vi "Read ADU Packet.vi"(8 "error in":errorcluster, 10 "isMaster (f)":bool, 11 "IP simple ADU in":refnum<class "SMSD ADU.lvclass">) -> (0 "error out":errorcluster, 2 "SMSD data unit out":refnum<class "SMSD Data Unit.lvclass">, 3 "IP simple ADU out":refnum<class "SMSD ADU.lvclass">, 5 "PDU Valid?":bool)   [LabVIEW 2021, in "SMSD ADU.lvclass"]
doc: "This uses the protocol layer to read a modbus packet off of the bus, wrapped in the IP transmission data unit."
uses:
  SMSD ADU.lvclass
  Data Unit/SMSD Data Unit/SMSD Data Unit.lvclass
  SMSD ADU.lvclass/SMSD ADU.ctl
  Data Unit/SMSD Data Unit/SMSD Data Unit.lvclass/SMSD Data Unit.ctl
  <vilib>/Utility/error.llb/Clear Errors.vi
  Modbus_v121c/Network Interface/TCP Interface/TSC/TCP Shared Components.lvlib
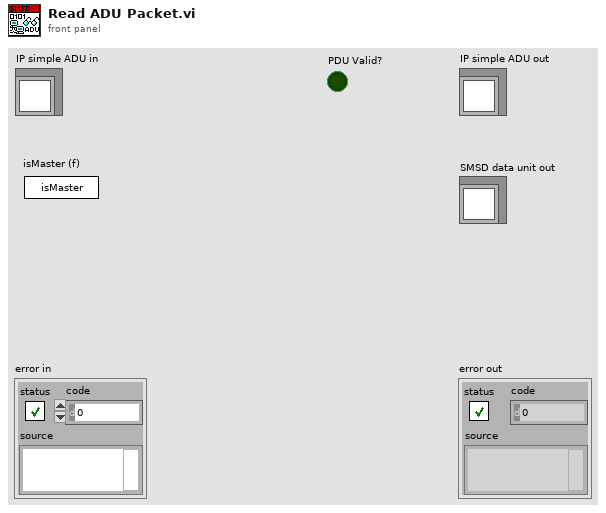
[diagram p1: front panel]
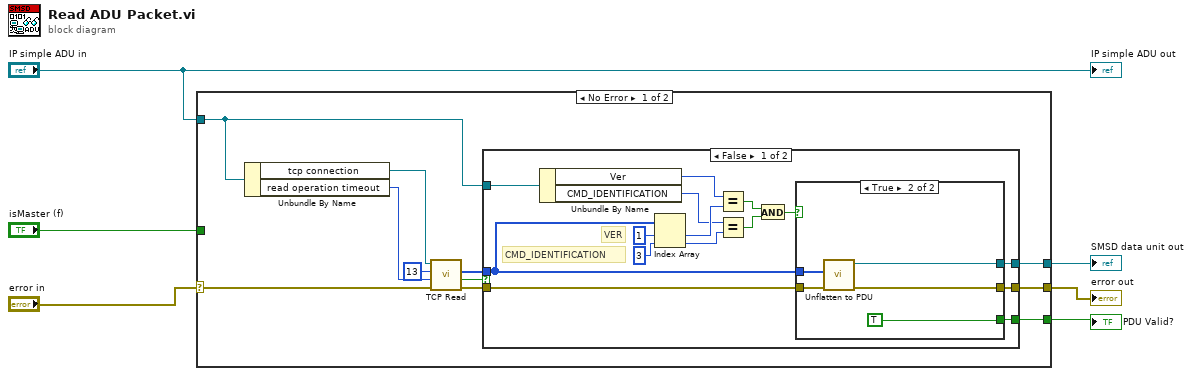
[diagram p0: block diagram]
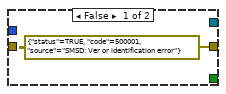
[diagram p2: hidden frame]
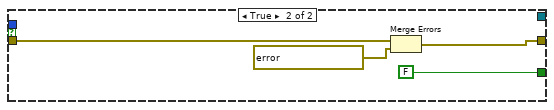
[diagram p3: hidden frame]
diagram:
  n1 = case shown="No Error" "error in" {
    selector: "error in" -> [w11 w43]
    tunnel: [w17 w43] -> w5
    tunnel: "IP simple ADU in" -> [w7 _]
    tunnel: [w16 _] -> w6
    tunnel: "isMaster (f)" -> [_ _]
    tunnel: [w9 _] -> w2
    frame No Error {
      n2 = Unbundle By Name(w7) -> ("tcp connection"=w12:refnum<k5>, "read operation timeout"=w10:u32)
      n3 = call "TCP Read.vi"("error in"=w11, "timeout"=w10, "bytes to read"=13, "connection ID"=w12) -> ("error out"=w15:errorcluster, "timed out?"=w14:bool, "data"=w13:u8[])  [unwired: 4 in, 1 out]
      n4 = case shown="False" w14 {
        tunnel: w15 -> [w31 w41]
        tunnel: [w30 w42] -> w17
        tunnel: w13 -> [w27 _]
        tunnel: [w32 FALSE] -> w16
        tunnel: [w29 _] -> w9
        tunnel: w7 -> [w25 _]
        frame False {
          # "CMD_IDENTIFICATION"
          # "VER"
          n5 = Unbundle By Name(w25) -> ("Ver"=w24:u8, "CMD_IDENTIFICATION"=w22:u8)
          n6 = Index Array(array=w27, index #1=1 ("index"), index #2=3 ("index")) -> (element #1=w23:u8, element #2=w21:u8)
          n7 = Equal?(x=w24, y=w23) -> (x = y?=w20:bool)
          n8 = Equal?(x=w22, y=w21) -> (x = y?=w19:bool)
          n9 = And(x=w20, y=w19) -> (x .and. y?=w18:bool)
          n10 = case shown="True" w18 {
            tunnel: [_ TRUE] -> w32
            tunnel: w31 -> [_ w37]
            tunnel: [errorcluster {"status"=TRUE, "code"=500001, "source"="SMSD: Ver or identification error"} ("error out") w36] -> w30
            tunnel: [_ w35] -> w29
            tunnel: w27 -> [_ w34]
            frame False {
            }
            frame True {
              n11 = call "Unflatten to PDU.vi"("error in"=w37, "SMSD data unit data"=w34) -> ("error out"=w36:errorcluster, "modbus data unit out"=w35:refnum<class "SMSD Data Unit.lvclass">)  [unwired: 8 in]
            }
          }
        }
        frame True {
          n12 = Merge Errors(w41, errorcluster {"status"=TRUE, "code"=56, "source"="LabVIEW: The network operation exceeded the user-specified or system time limit"} ("error out")) -> (w42:errorcluster)
        }
      }
    }
    frame Error {
    }
  }
  "error out" <- w5
  "PDU Valid?" <- w6
  "SMSD data unit out" <- w2
  "IP simple ADU out" <- "IP simple ADU in"
